vi "BRig_dataLC_Cue_First_DelayOpt_l1.vi"() -> (2 "output_Cue_First_DelayOpt":i32)   [LabVIEW 2014]
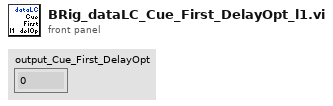
[diagram p1: front panel]
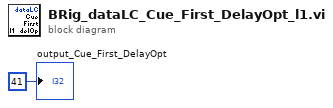
[diagram p0: block diagram]
diagram:
  "output_Cue_First_DelayOpt" <- 41 ("output_iBlock")
